vi "ex_subFileWrite.vi"(0 "Signals":dynamicdata(waveform), 1 "error in (no error)":errorcluster, 3 "Comment":string, 4 "Enable":bool=TRUE, 6 "new_file":bool, 7 "File Path in":path=path "c:/testdata.txt", 8 "File Dialog":bool, 9 "column headings":enum32{"one per segment", "once", "none"}(radio), 10 "Description":string, 11 "x_columns":enum32{"none", "one", "multiple"}(radio)=enum."multiple", 12 "multi_file":bool, 13 "fixed_width":bool=TRUE, 14 "serno_digits":i32=3, 15 "time_format_string":string="%Y-%m-%d_%H%M%S", 16 "overwrite_mode_multi":T6(ring)=enum."overwrite & backup", 17 "new_file_mode":u16(ring)=1 items=["Date & Time", "Serial No.", "Both"], 18 "overwrite_mode":T1(radio)=enum."overwrite & backup", 19 "new file options":T5, 20 "delimiter":string="\t", 22 "Reset":bool, 23 "Static File Path in":path=path "c:/testdata.txt", 24 "Lock file":bool, 25 "Simulate Non-First Call":bool, 26 "storage_format":T2, 27 "Ask each iteration":bool) -> (2 "error out":errorcluster, 5 "File Path out":path, 21 "Saving Data":bool)   [LabVIEW 2017]
uses:
  <vilib>/express/express output/ExFileWriteBlock.llb/ex_NewFileOptions.ctl
  <vilib>/express/express output/ExFileWriteBlock.llb/ex_WriteFileParams.ctl
  <vilib>/express/express input/ExFileReadBlock.llb/ex_ReadFileParams.ctl
  <vilib>/express/express shared/ExFile.llb/ex_FileFormats.ctl
panel:
  out "previous path":path
  in  "file params":T3={"delimiter"="\t", "origin time"=timestamp(0 s since 1904-01-01), "Flags"={"include col headings?"=TRUE, "x_columns"=0, "col headings always?"=TRUE, "time preference"=0, "hide col headings"=FALSE}, "Decimal Separator"=""} {"Flags"."time preference" items=["Absolute", "Relative"]; "Flags"."x_columns" items=["None", "One", "Multiple"]; "origin time" format="%<%X\n%x>T"}
  in  "1st":bool
  in  "File refnum":refnum<file>
  in  "origin time":timestamp format="%<%I:%M:%S %p\n%m/%d/%Y>T"
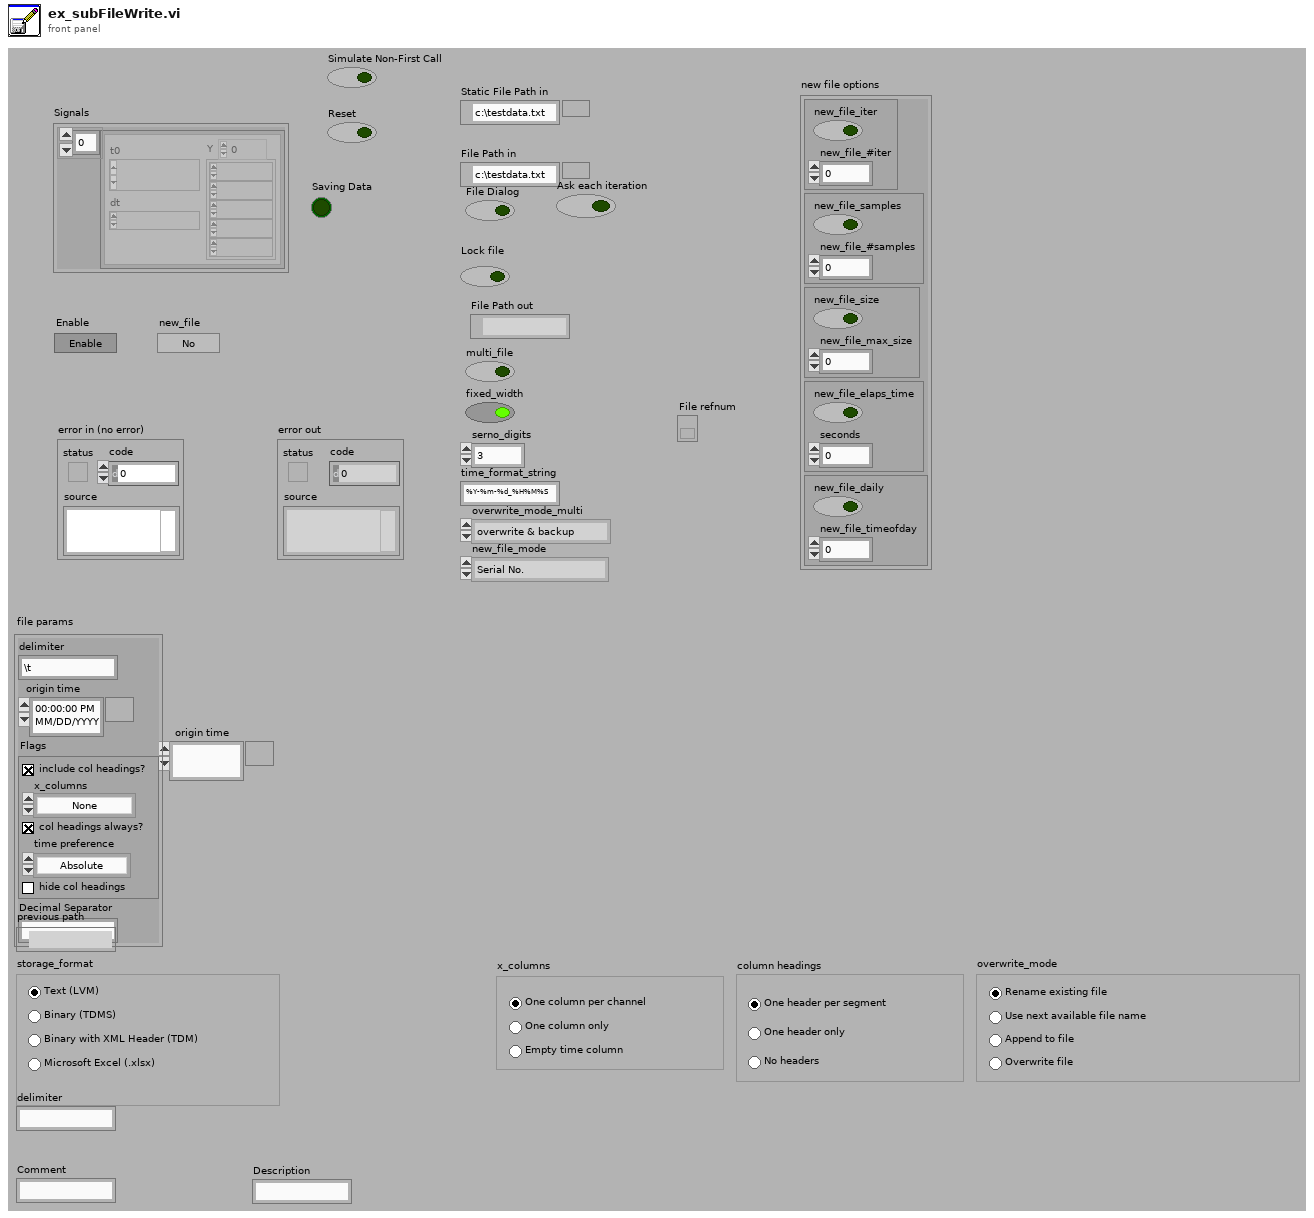
[diagram p1: front panel]
types:
  T1 = enum32{"overwrite", "overwrite & backup", "append", "next avail"}
  T2 = typedef "ex_FileFormats.ctl" = enum32{"lvm", "tdm", "tdms", "xlsx"}
  T3 = typedef "ex_WriteFileParams.ctl" = cluster{"delimiter":string, "origin time":timestamp, "Flags":T4, "Decimal Separator":string}
  T4 = typedef "ex_ReadFileParams.ctl" = cluster{"include col headings?":bool, "x_columns":u16, "col headings always?":bool, "time preference":u16, "hide col headings":bool}
  T5 = typedef "ex_NewFileOptions.ctl" = cluster{cluster{"new_file_iter":bool, "new_file_#iter":i32}, cluster{"new_file_samples":bool, "new_file_#samples":i32}, cluster{"new_file_size":bool, "new_file_max_size":i32}, cluster{"new_file_elaps_time":bool, "seconds":i32}, cluster{"new_file_daily":bool, "new_file_timeofday":i32}}
  T6 = enum16{"overwrite", "overwrite & backup", "next avail"}
  T7 = typedef "ex_userdefproperties.ctl" = cluster{"DAQmx Task":refnum<k21>, "User-defined properties":T8[], "Live values":variant[]}
  T8 = typedef "ex_userDefProperty.ctl" = cluster{"Name":string, "Object type":string, "usiDataType":T9, "propertySourceType":T10, "propertySource":string, "Value":variant, "ID":i32, "use def name":bool, "Source":string, "Built-in Prop":bool, "Attribute Type Enum":string[]}
  T9 = typedef "usiDataType.ctl" = enum16{"eNoTypeUsi", "eInt8Usi", "eInt16Usi", "eInt32Usi", "eInt64Usi", "eUInt8Usi", "eUInt16Usi", "eUInt32Usi", "eUInt64Usi", "eFloat32Usi", "eFloat64Usi", "- 0", "- 1", "- 2", "- 3", "- 4", "- 5", "- 6", "- 7", "- 8", "- 9", "eString8Usi", "eString16Usi", "eStringUsi", "eEnumUsi", "- 10", "- 11", "- 12", "- 13", "- 14", "eTimeUsi", "- 15", "- 16", "- 17", "- 18", "- 19", "- 20", "- 21", "- 22", "- 23", "eInstanceUsi", "eStoreUsi"}
  T10 = typedef "ex_propertySource.ctl" = enum16{"Manual", "System", "DAQmx Channel", "Terminal", "Ignore"}
  T11 = cluster{"file params":T3, "column headings":enum32{"one per segment", "once", "none"}, "origin time":timestamp, "File refnum":refnum<file>, "overwrite_mode_multi":enum16{"overwrite", "overwrite & backup", "next avail"}, "overwrite_mode":enum32{"overwrite", "overwrite & backup", "append", "next avail"}, "File Dialog":bool, "Description Out":string, "Comment Out":string, "serno_digits":i32, "fixed_width":bool, "new_file_mode":u16, "time_format_string":string, "multi_file":bool, "new file options":T5, "new_file":bool, "Simulate Non-First Call":bool}
  T12 = cluster{"channel\nrefnums":refnum<k20>[], "channel names":string[], "channel types":string[], "file refnum":refnum<k20>, "group refnum":refnum<k20>, "group name":string, "group type":string, "next T0":timestamp[], "dT":dbl[], "Start Time Stamp":timestamp, "channel length":u32[], "group index":u32, "group refnums":refnum<k20>[], "file name":string, "segment index":u32}
  T13 = typedef "ex_appendInfoTDM.ctl" = cluster{"channel\nrefnums":refnum<k20>[], "channel names":string[], "channel types":string[], "file refnum":refnum<k20>, "group refnum":refnum<k20>, "group name":string, "group type":string, "next T0":timestamp[], "dT":dbl[], "Start Time Stamp":timestamp, "channel length":u32[], "group index":u32, "group refnums":refnum<k20>[], "file name":string, "segment index":u32}
  T14 = cluster{"Start Timestamp":timestamp, "Timestamp":timestamp, "Relative Time?":bool, "X Dimension":string, "Signal Name":string, "Y Units":string, "X0":timestamp, "dX":dbl, "nPoints":i32}[]
  T15 = typedef "ex_WaveformAttribsPlus.ctl" = cluster{"Start Timestamp":timestamp, "Timestamp":timestamp, "Relative Time?":bool, "X Dimension":string, "Signal Name":string, "Y Units":string, "X0":timestamp, "dX":dbl, "nPoints":i32}
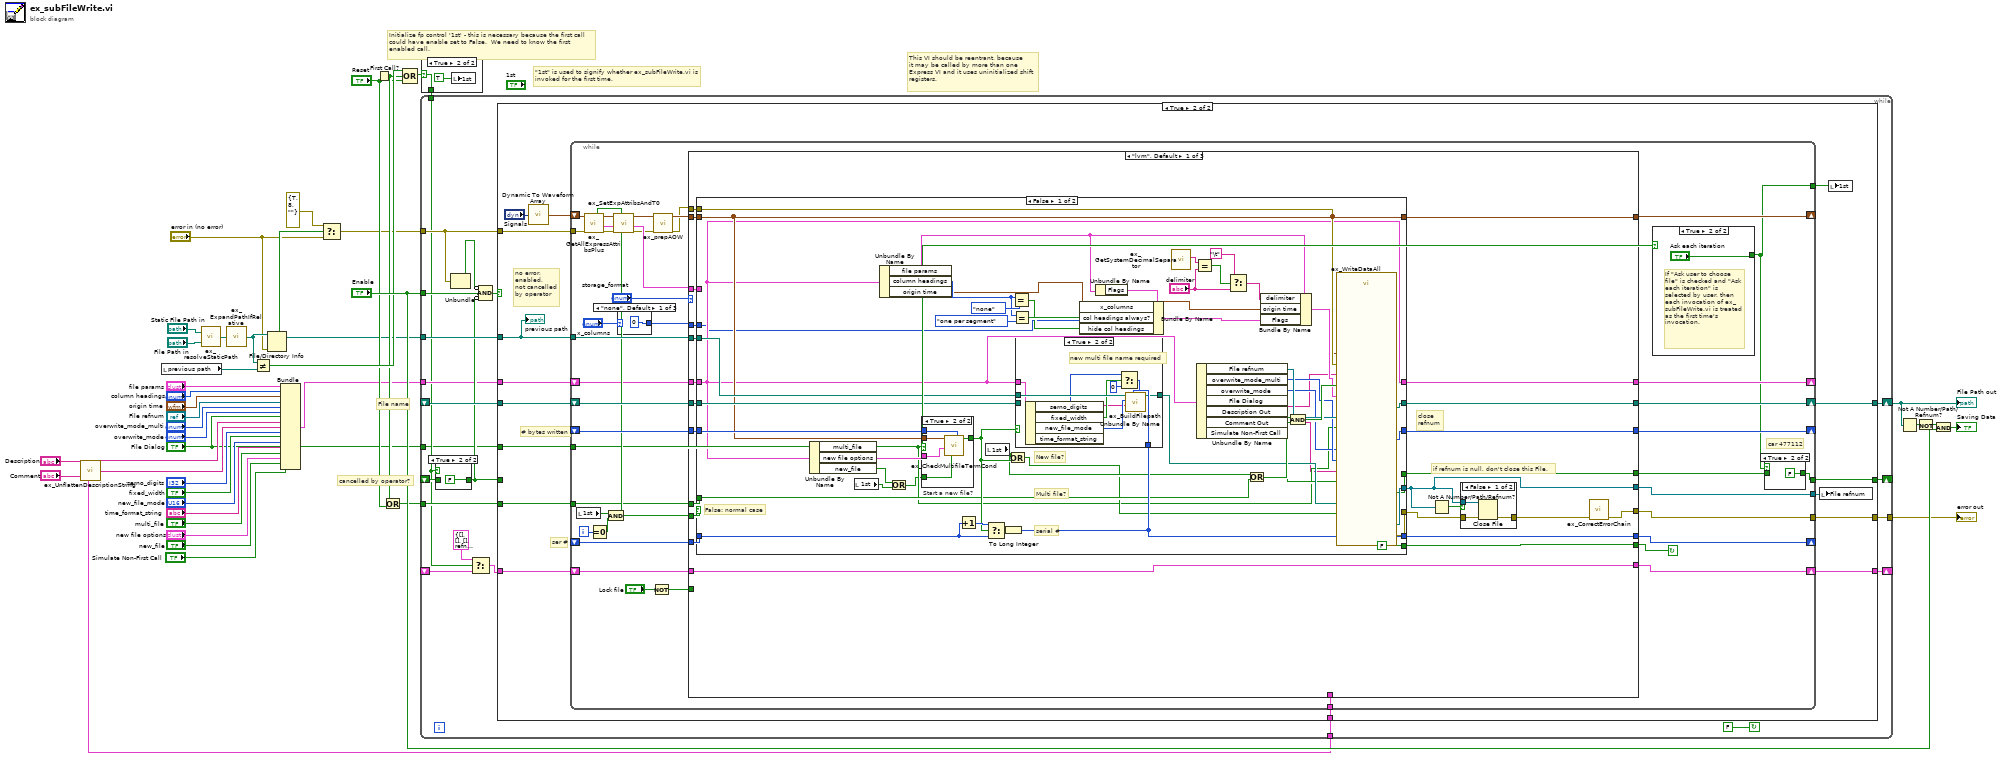
[diagram p0: block diagram]
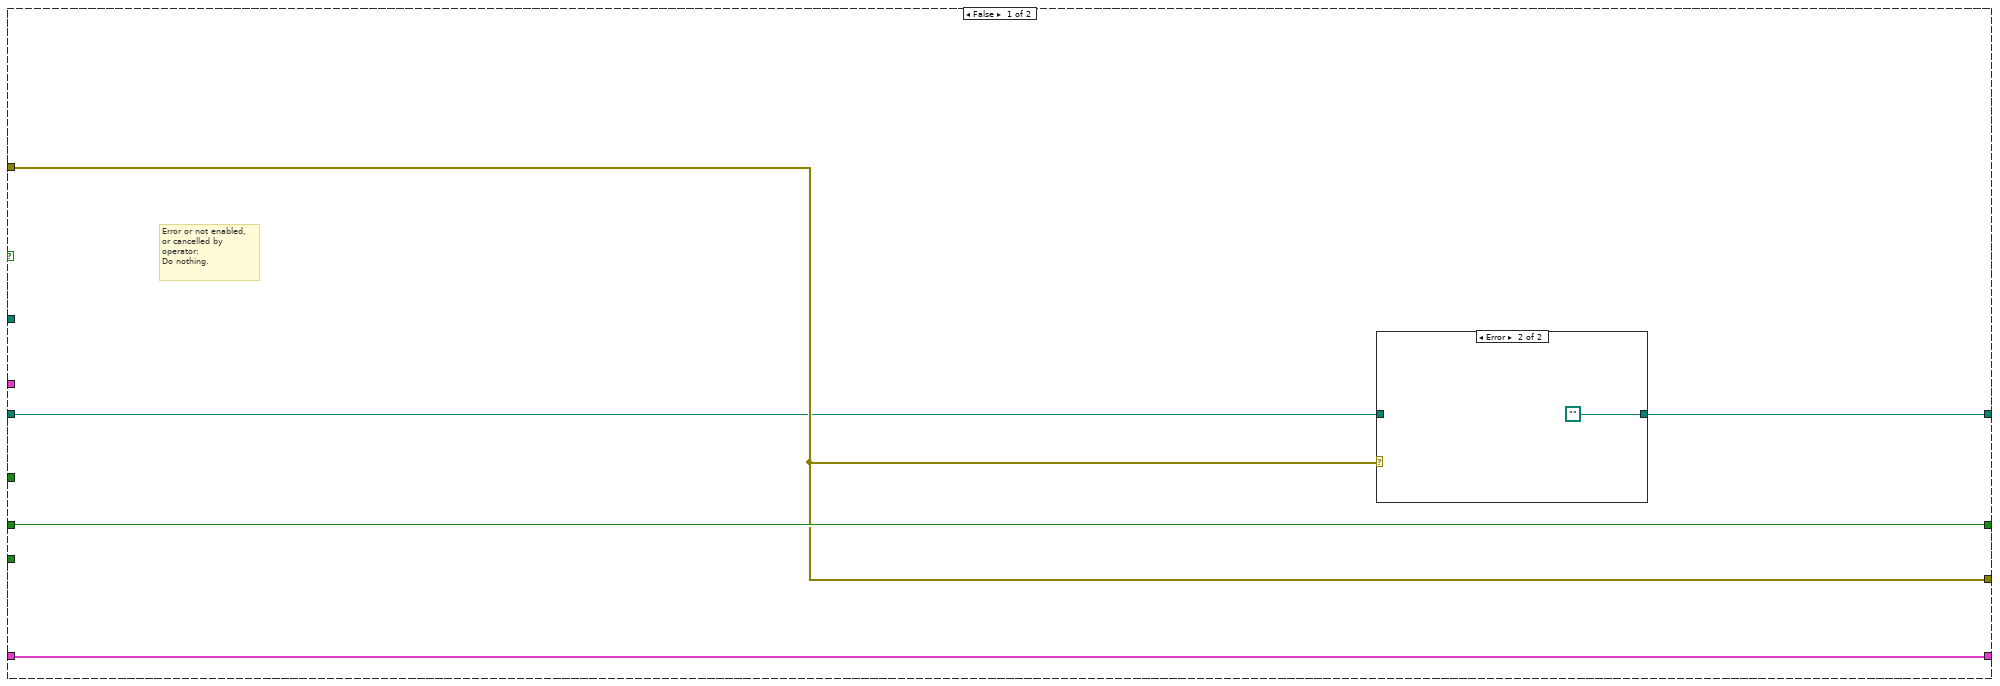
[diagram p3: hidden frame]
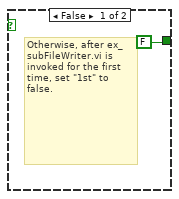
[diagram p6: hidden frame]
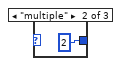
[diagram p7: hidden frame]
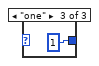
[diagram p8: hidden frame]
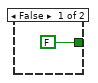
[diagram p11: hidden frame]
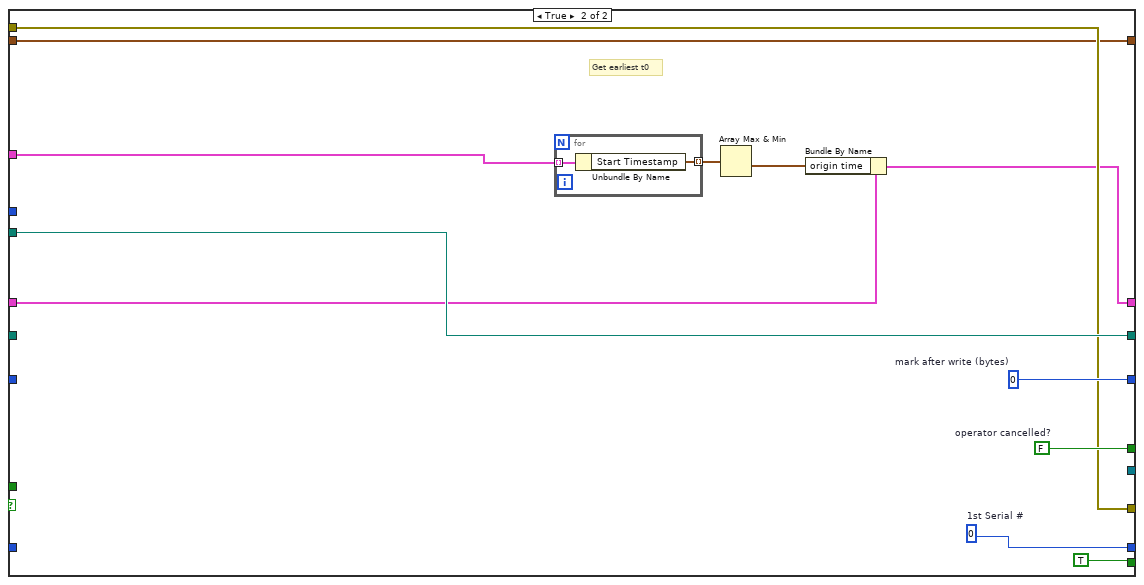
[diagram p12: hidden frame]
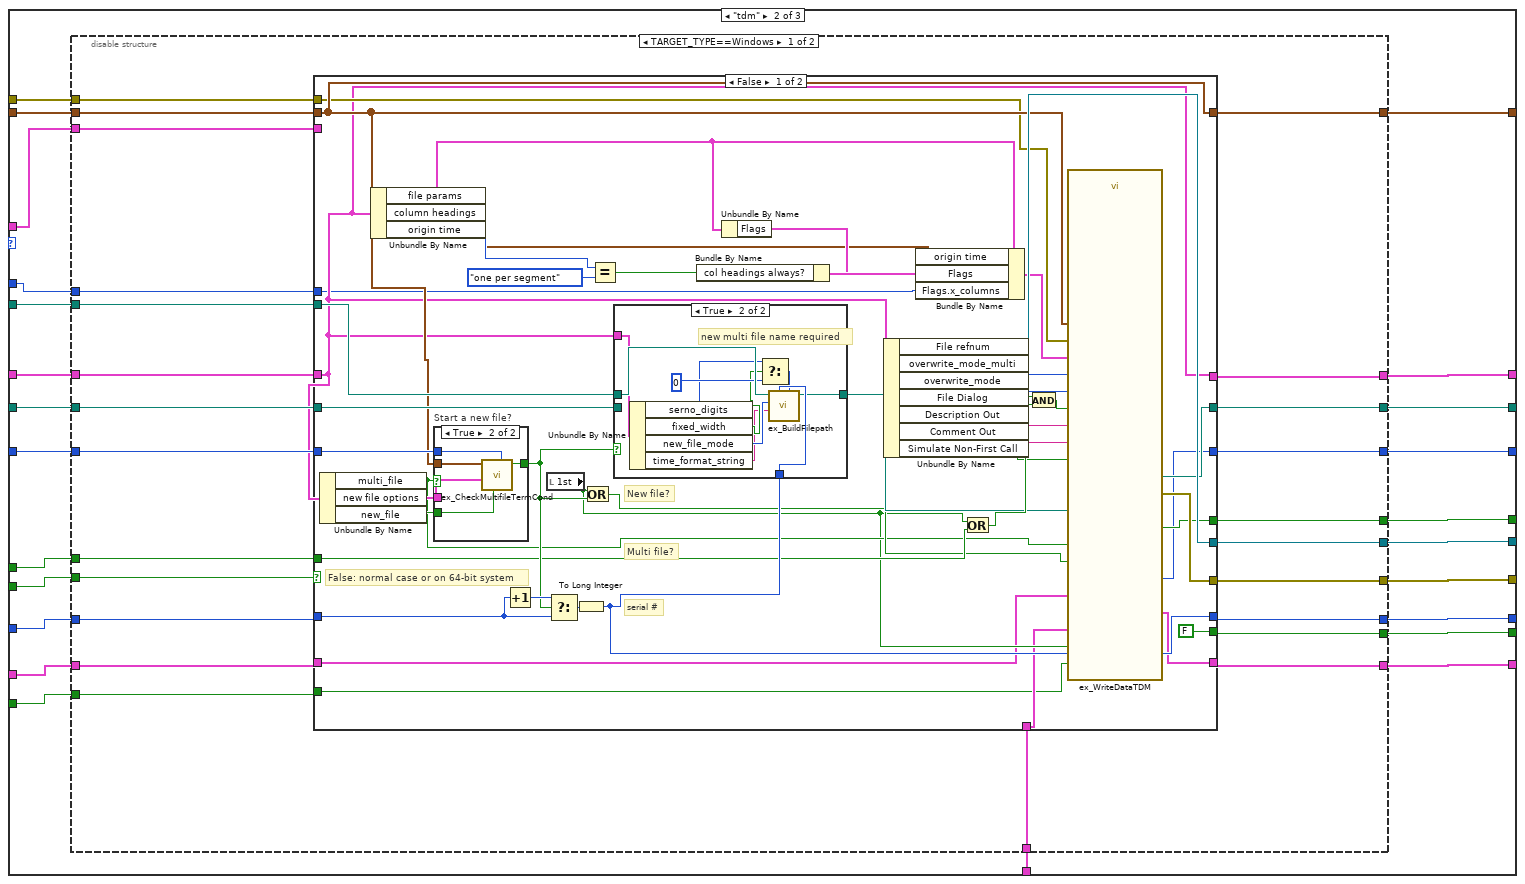
[diagram p13: hidden frame]
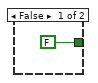
[diagram p15: hidden frame]
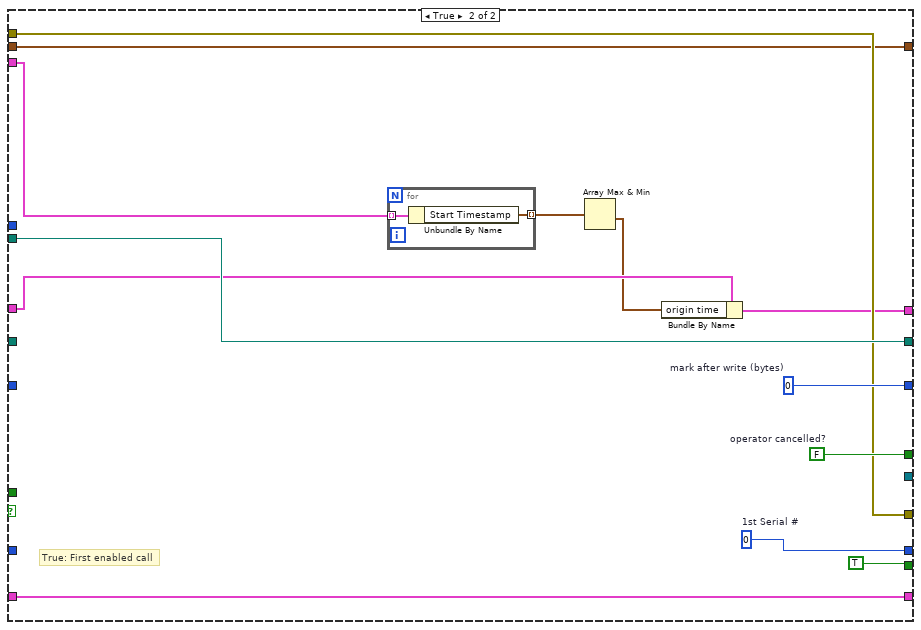
[diagram p16: hidden frame]
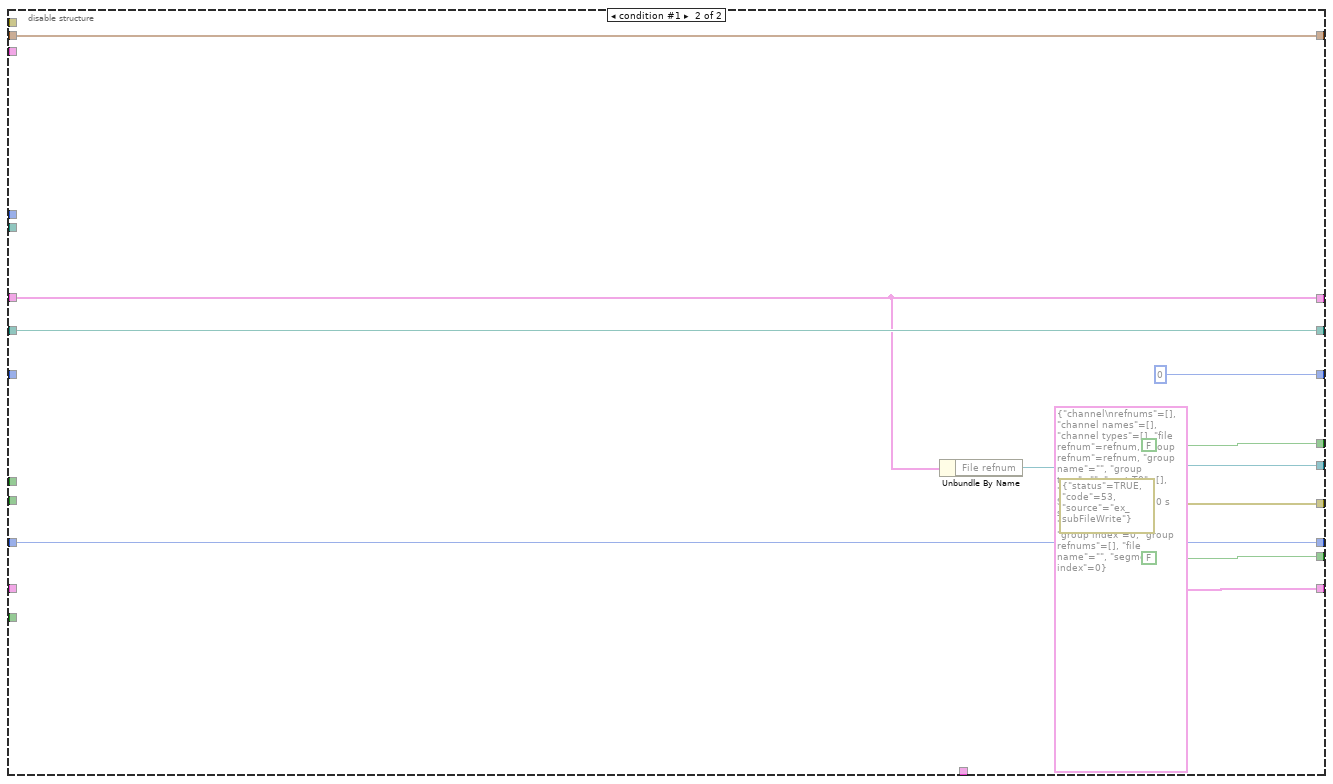
[diagram p17: hidden frame]
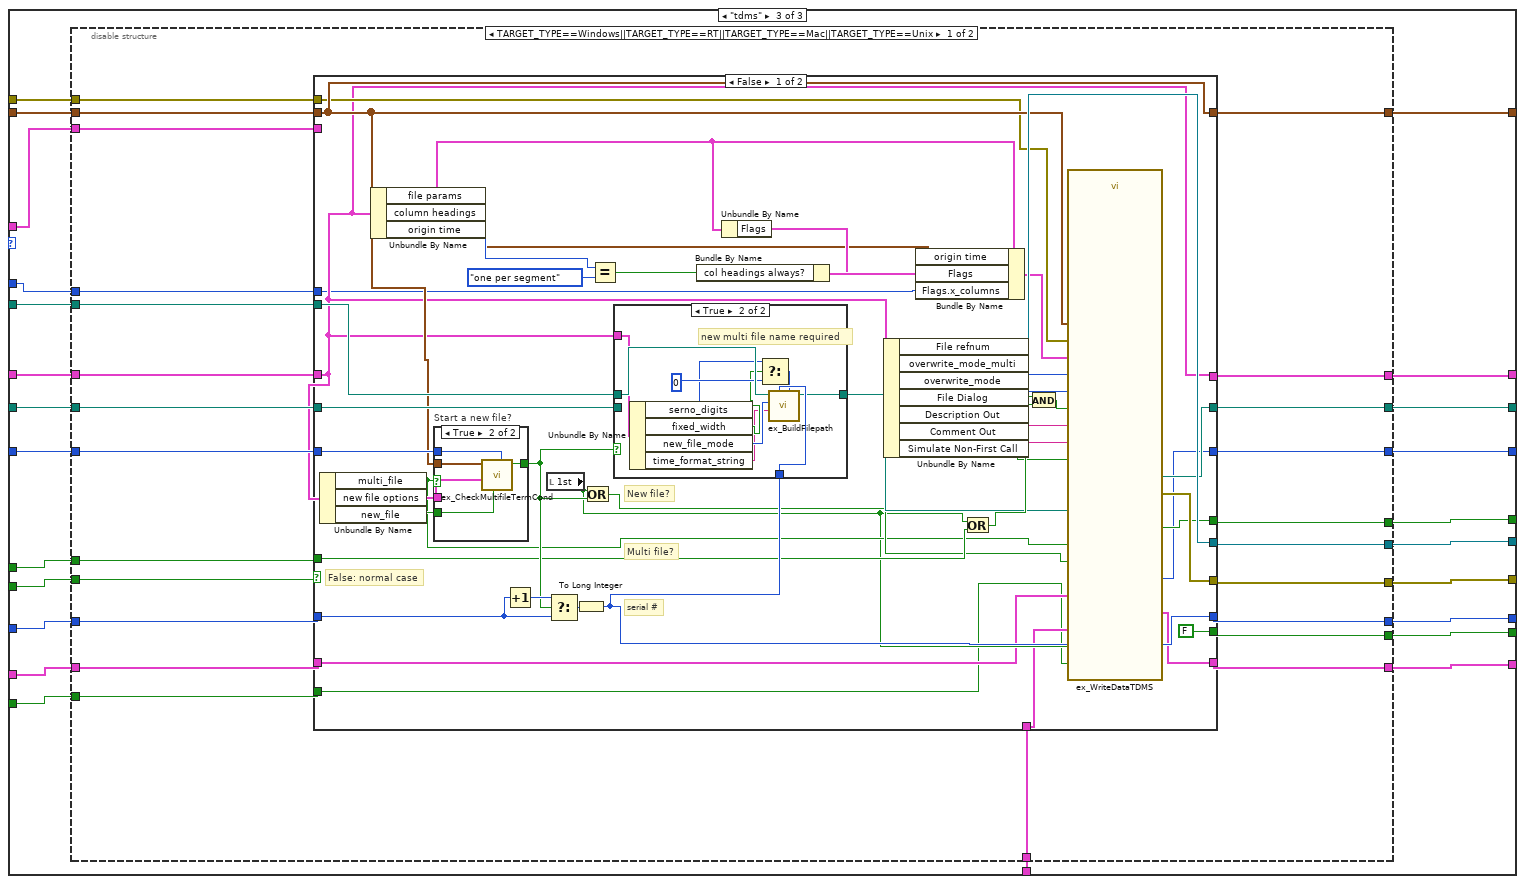
[diagram p18: hidden frame]
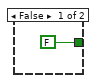
[diagram p20: hidden frame]
diagram:
  # "\"1st\" is used to signify whether ex_subFileWrite.vi is invoked for the first time."
  # "File name"
  # "This VI should be reentrant, because\nit may be called by more than one\nExpress VI and it uses uninitialized shift \nregisters."
  # "cancelled by operator?"
  # "Initialize fp control '1st' - this is necessary because the first call\ncould have enable set to False.  We need to know the first\nenabled call."
  n1 = call <vilib>:"ex_UnflattenDescriptionString.vi"("Description"="Description", "Comment"="Comment") -> ("Description Out"=w6:string, "Comment Out"=w5:string, "DAQmx Task"=w4:T7)
  n2 = local read "previous path"() -> (w36:path)
  n3 = call <vilib>:"ex_resolveStaticPath.vi"("file path in"="File Path in", "static path in"="Static File Path in") -> ("Path"=w13:path)
  n4 = call <vilib>:"ex_ExpandPathIfRelative.vi"("Path"=w13) -> ("Expanded path"=w12:path)  [unwired: 4 out]
  n5 = Not Equal?(x=w12, y=w36) -> (x != y?=w34:bool)
  n6 = File/Directory Info(path=w12, error in="error in (no error)") -> (path out=w11:path, directory=w9:bool)  [unwired: 5 out]
  n7 = Bundle("file params"="file params", "column headings"="column headings", "origin time"="origin time", "File refnum"="File refnum", "overwrite_mode_multi"="overwrite_mode_multi", "overwrite_mode"="overwrite_mode", "File Dialog"="File Dialog", "Description Out"=w6, "Comment Out"=w5, "serno_digits"="serno_digits", "fixed_width"="fixed_width", "new_file_mode"="new_file_mode", "time_format_string"="time_format_string", "multi_file"="multi_file", "new file options"="new file options", "new_file"="new_file", "Simulate Non-First Call"="Simulate Non-First Call") -> (w14:T11)  [unwired: 1 out]
  n8 = Select(t=errorcluster {"status"=TRUE, "code"=8, "source"=""}, s=w9, f="error in (no error)") -> (s? t:f=w10:errorcluster)
  n9 = First Call?() -> (First Call?: T/F=w33:bool)
  n10 = Or(x=w33, y="Reset") -> (x .or. y?=w31:bool)
  n11 = Compound Arithmetic op=OR(w34, w33, "Reset") -> (w35:bool)
  n12 = case shown="False" w35 {
    selector: w35 -> [w44 w45]
    tunnel: [w44 w45] -> w43
    frame False {
    }
    frame True {
      n13 = local write "1st"(TRUE ("1st")) -> ()
    }
  }
  n14 = while {
    tunnel: [w67] -> w30
    tunnel: w43 -> [w48]
    tunnel: w10 -> [w65]
    shift-right: [w63] -> _
    shift-left: _ -> [w62]
    shift-right: [w60] -> w29
    shift-left: _ -> [w61]
    tunnel: "Enable" -> [w59]
    tunnel: w11 -> [w58]
    tunnel: w31 -> [w55]
    tunnel: w14 -> [w54]
    shift-right: [w53] -> _
    shift-left: _ -> [w50]
    tunnel: w4 -> [w52]
    tunnel: "File Dialog" -> [w47]
    stop <- FALSE continue-if-true
    n15 = case shown="True" w48 {
      tunnel: w62 -> [w68 _]
      tunnel: [w68 FALSE ("operator cancelled?")] -> w56
      frame False {
      }
      frame True {
      }
    }
    n16 = Unbundle(w65) -> ("status"=w57:bool)  [unwired: 2 out]
    n17 = Select(t=T12 {"channel\nrefnums"=[], "channel names"=[], "channel types"=[], "file refnum"=refnum, "group refnum"=refnum, "group name"="", "group type"="", "next T0"=[], "dT"=[], "Start Time Stamp"=timestamp(0 s since 1904-01-01), "channel length"=[], "group index"=0, "group refnums"=[], "file name"="", "segment index"=0} ("append info out"), s=w48, f=w50) -> (s? t:f=w49:T13)
    n18 = Compound Arithmetic op=AND(invert w57, w59, invert w56) -> (w66:bool)
    n19 = case shown="True" w66 {
      tunnel: [w72 w83] -> w67
      tunnel: w65 -> [w72 w92]
      tunnel: [w74 w91] -> w63
      tunnel: w56 -> [w74 _]
      tunnel: [w71 w90] -> w60
      tunnel: w61 -> [w70 w89]
      tunnel: w58 -> [_ w80]
      tunnel: w55 -> [_ w87]
      tunnel: w54 -> [_ w85]
      tunnel: [w73 w82] -> w53
      tunnel: w49 -> [w73 w81]
      tunnel: w52 -> [_ w79]
      tunnel: w47 -> [_ w77]
      frame False {
        # "Error or not enabled,\nor cancelled by\noperator:\nDo nothing."
        n20 = case shown="No Error" w72 {
          tunnel: [w75 path ""] -> w71
          tunnel: w70 -> [w75 _]
          frame No Error {
          }
          frame Error {
          }
        }
      }
      frame True {
        # "no error,\nenabled,\nnot cancelled\nby operator"
        # "# bytes written"
        # "ser #"
        n21 = call <vilib>:"Dynamic To Waveform Array.vi"("Input"="Signals") -> ("Output"=w84:waveform(dbl)[])  [unwired: 4 out]
        n22 = while {
          tunnel: w92 -> [w121]
          shift-right: [w130] -> _
          shift-left: _ -> [w129]
          tunnel: [w132] -> w83
          shift-right: [w122] -> w90
          shift-left: w89 -> [w128]
          shift-right: [w124] -> _
          shift-left: _ -> [w131]
          tunnel: [w127] -> w86
          tunnel: w80 -> [w123]
          tunnel: [w93] -> w91
          shift-right: [w120] -> _
          shift-left: w84 -> [w109]
          tunnel: w87 -> [w112]
          shift-right: [w108] -> _
          shift-left: w85 -> [w110]
          shift-right: [w107] -> w82
          shift-left: w81 -> [w106]
          tunnel: w79 -> [w99]
          tunnel: [w95] -> w78
          tunnel: w77 -> [w96]
          i -> [w126]
          stop <- w133 continue-if-true
          # "car 477112"
          n23 = local read "1st"() -> (w113:bool)
          n24 = call <vilib>:"ex_GetAllExpressAttribsPlus.vi"("error in"=w121, "Signals in"=w109) -> ("error out"=w115:errorcluster, "All Express Wave Attributes Plus"=w114:T14, "Signals out"=w118:waveform(dbl)[], "Time Attribs Not Found"=w116:bool[])  [unwired: 1 in, 5 out]
          n25 = Equal To 0?(x=w126) -> (x = 0?=w125:bool)
          n26 = And(x=w113, y=w125) -> (x .and. y?=w119:bool)
          n27 = call <vilib>:"ex_SetExpAttribsAndT0.vi"("Latch Origin TS? (T)"=w119, "Set? (T if empty)"=w116, "error in (no error)"=w115, "Express Attributes Plus in"=w114, "Signals"=w118) -> ("error out"=w101:errorcluster, "Express Wave Attributes Plus out"=w117:T15[], "Signals With Attributes"=w103:waveform(dbl)[])  [unwired: 1 in, 3 out]
          n28 = case shown="\"none\", Default" "x_columns" {
            tunnel: [u16 0 ("x_columns") u16 2 ("x_columns") u16 1 ("x_columns")] -> w104
            frame "none", Default {
            }
            frame "multiple" {
            }
            frame "one" {
            }
          }
          n29 = Not(x="Lock file") -> (.not. x?=w97:bool)
          n30 = call <vilib>:"ex_prepAOW.vi"("error in (no error)"=w101, "Dynamic Data"=w103) -> ("error out"=w100:errorcluster, 3:w102:waveform(dbl)[])  [unwired: 1 in, 3 out]
          n31 = case shown="\"lvm\", Default" "storage_format" {
            tunnel: [w164 w274 w409] -> w133
            tunnel: [w148 w273 w408] -> w132
            tunnel: w131 -> [w163 w272 w407]
            tunnel: [w162 w271 w406] -> w130
            tunnel: w129 -> [w161 w270 w405]
            tunnel: w128 -> [w160 w269 w404]
            tunnel: [w141 w258 w393] -> w127
            tunnel: [w159 w268 w403] -> w124
            tunnel: w123 -> [w158 w267 w402]
            tunnel: [w157 w266 w401] -> w94
            tunnel: [w156 w265 w400] -> w122
            tunnel: [w155 w264 w399] -> w120
            tunnel: w119 -> [w154 w263 w398]
            tunnel: w102 -> [w153 w257 w392]
            tunnel: w100 -> [w152 w262 w397]
            tunnel: w117 -> [w151 w261 w396]
            tunnel: w112 -> [w150 w260 w395]
            tunnel: w110 -> [w149 w259 w394]
            tunnel: [w147 w256 w391] -> w108
            tunnel: [w146 w255 w390] -> w107
            tunnel: w106 -> [w146 w254 w389]
            tunnel: w104 -> [w145 w253 w388]
            tunnel: w99 -> [_ w252 w387]
            tunnel: w97 -> [_ w251 w386]
            frame "lvm", Default {
              # "if refnum is null, don't close this File."
              # "close\nrefnum"
              n32 = case shown="False" w154 {
                tunnel: [FALSE TRUE] -> w164
                tunnel: [w192 _] -> w141
                tunnel: [w189 w241] -> w144
                tunnel: [w190 w248] -> w159
                tunnel: w163 -> [w212 _]
                tunnel: w152 -> [w208 w241]
                tunnel: [w217 w246] -> w162
                tunnel: [w191 w247] -> w156
                tunnel: w161 -> [w218 _]
                tunnel: w160 -> [w214 _]
                tunnel: w153 -> [w182 w240]
                tunnel: w158 -> [w211 w247]
                tunnel: [w183 w244] -> w157
                tunnel: w151 -> [_ w242]
                tunnel: [w182 w240] -> w155
                tunnel: w150 -> [w201 _]
                tunnel: w149 -> [w180 w239]
                tunnel: [w180 w237] -> w147
                tunnel: w145 -> [w179 _]
                frame False {
                  # "Multi file?"
                  # "New file?"
                  # "False: normal case"
                  # "serial #"
                  n33 = Unbundle By Name(w180) -> ("multi_file"=w184:bool, "new file options"=w193:T5, "new_file"=w171:bool)
                  n34 = local read "1st"() -> (w170:bool)
                  n35 = Unbundle By Name(w180) -> ("file params"=w199:T3, "column headings"=w198:enum32{"one per segment", "once", "none"}, "origin time"=w181:timestamp)
                  n36 = Or(x=w171, y=w170) -> (x .or. y?=w169:bool)
                  n37 = case "Start a new file?" shown="True" w184 {
                    tunnel: [FALSE ("start new file?") w236] -> w213
                    tunnel: w182 -> [_ w235]
                    tunnel: w212 -> [_ w234]
                    tunnel: w193 -> [_ w233]
                    tunnel: w169 -> [_ w232]
                    frame False {
                    }
                    frame True {
                      n38 = call <vilib>:"ex_CheckMultifileTermCond.vi"("file size (bytes)"=w234, "new_file_now"=w232, "termination conditions"=w233, "Signals"=w235) -> ("start new file?"=w236:bool)  [unwired: 7 out]
                    }
                  }
                  n39 = Increment(x=w218) -> (x+1=w219:i32)
                  n40 = local read "1st"() -> (w200:bool)
                  n41 = Select(t=w219, s=w213, f=w218) -> (s? t:f=w216:i32)
                  n42 = To Long Integer(number=w216) -> (32bit integer=w217:i32)
                  n43 = Or(x=w200, y=w213) -> (x .or. y?=w185:bool)
                  n44 = Equal?(x=w198, y=enum16{"one per segment", "once", "none"}."none") -> (x = y?=w204:bool)
                  n45 = Equal?(x=w198, y=enum16{"one per segment", "once", "none"}."one per segment") -> (x = y?=w205:bool)
                  n46 = case shown="True" w213 {
                    tunnel: w217 -> [_ w230]
                    tunnel: [w220 w229] -> w188
                    tunnel: w214 -> [w220 _]
                    tunnel: w211 -> [_ w228]
                    tunnel: w180 -> [_ w225]
                    frame False {
                      # "No new file - use old file name"
                    }
                    frame True {
                      # "new multi file name required"
                      n47 = Unbundle By Name(w225) -> ("serno_digits"=w224:i32, "fixed_width"=w223:bool, "new_file_mode"=w222:u16, "time_format_string"=w221:string)
                      n48 = Select(t=w224, s=w223, f=0) -> (s? t:f=w226:i32)
                      n49 = call <vilib>:"ex_BuildFilepath.vi"("serial digits"=w226, "serial num"=w230, "time format string"=w221, "naming mode"=w222, "name base"=w228) -> ("built name"=w229:path)  [unwired: 1 in, 5 out]
                    }
                  }
                  n50 = Unbundle By Name(w199) -> ("Flags"=w209:T4)
                  n51 = Bundle By Name(cluster=w209, "x_columns"=w179, "col headings always?"=w205, "hide col headings"=w204) -> (w210:T4)
                  n52 = call <vilib>:"ex_GetSystemDecimalSeparator.vi"() -> ("Decimal Seperator"=w176:string)  [unwired: 11 out]
                  n53 = Equal?(x=w176, y="delimiter") -> (x = y?=w175:bool)
                  n54 = Unbundle By Name(w180) -> ("File refnum"=w197:refnum<file>, "overwrite_mode_multi"=w196:T6, "overwrite_mode"=w195:T1, "File Dialog"=w194:bool, "Description Out"=w177:string, "Comment Out"=w178:string, "Simulate Non-First Call"=w187:bool)
                  n55 = Select(t="\t", s=w175, f="delimiter") -> (s? t:f=w172:string)
                  n56 = Or(x=w200, y=w201) -> (x .or. y?=w203:bool)
                  n57 = Bundle By Name(cluster=w199, "delimiter"=w172, "origin time"=w181, "Flags"=w210) -> (w186:T3)
                  n58 = And(x=w194, y=w203) -> (x .and. y?=w202:bool)
                  n59 = call <vilib>:"ex_WriteDataAll.vi"("file path"=w188, "File refnum in"=w197, "Signals"=w182, "overwrite_mode_multi"=w196, "overwrite_mode"=w195, "error in (no error)"=w208, "file dialog?"=w202, "Description"=w177, "multi_file"=w184, "Comment"=w178, "new file?"=w185, "Simulate Non-First Call"=w187, "file params"=w186) -> ("operator cancelled?"=w183:bool, "file path out"=w191:path, "refnum out"=w192:refnum<file>, "mark after write (bytes)"=w190:i32, "error out"=w189:errorcluster)  [unwired: 2 out]
                }
                frame True {
                  w244 = FALSE  # operator cancelled?
                  w248 = 0  # mark after write (bytes)
                  w246 = 0  # 1st Serial #
                  # "True: First enabled call"
                  # "Get earliest t0"
                  n60 = for {
                    tunnel: w242 -> [w250] mode=indexing
                    tunnel: [w249] -> w243 mode=indexing
                    n61 = Unbundle By Name(w250) -> ("Start Timestamp"=w249:timestamp)
                  }
                  n62 = Array Max & Min(array=w243) -> (min value=w238:timestamp)  [unwired: 3 out]
                  n63 = Bundle By Name(cluster=w239, "origin time"=w238) -> (w237:T11)
                }
              }
              n64 = Not A Number/Path/Refnum?(number/path/refnum=w141) -> (NaN/Path/Refnum?=w142:bool)
              n65 = case shown="False" w142 {
                tunnel: w144 -> [w167 w168]
                tunnel: [w166 w168] -> w143
                tunnel: w141 -> [w165 _]
                frame False {
                  n66 = Close File(refnum=w165, error in=w167) -> (error out=w166:errorcluster)  [unwired: 1 out]
                }
                frame True {
                }
              }
              n67 = call <vilib>:"ex_CorrectErrorChain.vi"("error in (no error)"=w143) -> ("error out"=w148:errorcluster)  [unwired: 1 in, 9 out]
            }
            frame "tdm" {
              n68 = disable-structure shown="TARGET_TYPE==Windows" {
                disable-tunnel: [w298 FALSE] -> w274
                disable-tunnel: [w297 errorcluster {"status"=TRUE, "code"=53, "source"="ex_subFileWrite"} ("error out")] -> w273
                disable-tunnel: w272 -> [w296 _]
                disable-tunnel: [w295 w380] -> w271
                disable-tunnel: w270 -> [w294 w380]
                disable-tunnel: w269 -> [w293 w385]
                disable-tunnel: [w292 0 ("mark after write (bytes)")] -> w268
                disable-tunnel: w267 -> [w291 _]
                disable-tunnel: [w290 FALSE ("operator cancelled?")] -> w266
                disable-tunnel: [w289 w385] -> w265
                disable-tunnel: [w288 w384] -> w264
                disable-tunnel: w263 -> [w275 _]
                disable-tunnel: w262 -> [w287 _]
                disable-tunnel: w261 -> [w286 _]
                disable-tunnel: w260 -> [w276 _]
                disable-tunnel: w259 -> [w285 w383]
                disable-tunnel: [w284 w382] -> w258
                disable-tunnel: w257 -> [w283 w384]
                disable-tunnel: [w282 w383] -> w256
                disable-tunnel: [w281 T12 {"channel\nrefnums"=[], "channel names"=[], "channel types"=[], "file refnum"=refnum, "group refnum"=refnum, "group name"="", "group type"="", "next T0"=[], "dT"=[], "Start Time Stamp"=timestamp(0 s since 1904-01-01), "channel length"=[], "group index"=0, "group refnums"=[], "file name"="", "segment index"=0} ("append info out")] -> w255
                disable-tunnel: w254 -> [w280 _]
                disable-tunnel: w253 -> [w279 _]
                disable-tunnel: w252 -> [w278 _]
                disable-tunnel: w251 -> [w277 _]
                frame condition #0 (active) {
                  n69 = case shown="False" w275 {
                    tunnel: [FALSE TRUE] -> w298
                    tunnel: [w308 w368] -> w297
                    tunnel: [w306 w373] -> w292
                    tunnel: w296 -> [w336 _]
                    tunnel: w287 -> [w321 w368]
                    tunnel: [w341 w371] -> w295
                    tunnel: [w309 w372] -> w289
                    tunnel: w294 -> [w342 _]
                    tunnel: w293 -> [w338 _]
                    tunnel: w291 -> [w335 w372]
                    tunnel: [w307 w369] -> w290
                    tunnel: w286 -> [_ w366]
                    tunnel: [w322 w367] -> w288
                    tunnel: w276 -> [w329 _]
                    tunnel: w285 -> [w319 w364]
                    tunnel: [w323 _] -> w284
                    tunnel: w283 -> [w322 w367]
                    tunnel: [w319 w362] -> w282
                    tunnel: [w305 w361] -> w281
                    tunnel: w280 -> [w304 w361]
                    tunnel: w279 -> [w318 _]
                    tunnel: w278 -> [w303 _]
                    tunnel: w277 -> [w299 _]
                    frame False {
                      # "Multi file?"
                      # "New file?"
                      # "False: normal case or on 64-bit system"
                      # "serial #"
                      n70 = Unbundle By Name(w319) -> ("multi_file"=w311:bool, "new file options"=w325:T5, "new_file"=w324:bool)
                      n71 = Unbundle By Name(w319) -> ("file params"=w328:T3, "column headings"=w327:enum32{"one per segment", "once", "none"}, "origin time"=w320:timestamp)
                      n72 = case "Start a new file?" shown="True" w311 {
                        tunnel: [FALSE ("start new file?") w360] -> w337
                        tunnel: w322 -> [_ w359]
                        tunnel: w336 -> [_ w358]
                        tunnel: w325 -> [_ w357]
                        tunnel: w324 -> [_ w356]
                        frame False {
                        }
                        frame True {
                          n73 = call <vilib>:"ex_CheckMultifileTermCond.vi"("file size (bytes)"=w358, "new_file_now"=w356, "termination conditions"=w357, "Signals"=w359) -> ("start new file?"=w360:bool)  [unwired: 7 out]
                        }
                      }
                      n74 = Increment(x=w342) -> (x+1=w343:i32)
                      n75 = local read "1st"() -> (w310:bool)
                      n76 = Select(t=w343, s=w337, f=w342) -> (s? t:f=w340:i32)
                      n77 = To Long Integer(number=w340) -> (32bit integer=w341:i32)
                      n78 = Or(x=w310, y=w337) -> (x .or. y?=w312:bool)
                      n79 = Equal?(x=w327, y=enum16{"one per segment", "once", "none"}."one per segment") -> (x = y?=w331:bool)
                      n80 = case shown="True" w337 {
                        tunnel: w341 -> [_ w354]
                        tunnel: [w344 w353] -> w313
                        tunnel: w338 -> [w344 _]
                        tunnel: w335 -> [_ w352]
                        tunnel: w319 -> [_ w349]
                        frame False {
                          # "No new file - use old file name"
                        }
                        frame True {
                          # "new multi file name required"
                          n81 = Unbundle By Name(w349) -> ("serno_digits"=w348:i32, "fixed_width"=w347:bool, "new_file_mode"=w346:u16, "time_format_string"=w345:string)
                          n82 = Select(t=w348, s=w347, f=0) -> (s? t:f=w350:i32)
                          n83 = call <vilib>:"ex_BuildFilepath.vi"("serial digits"=w350, "serial num"=w354, "time format string"=w345, "naming mode"=w346, "name base"=w352) -> ("built name"=w353:path)  [unwired: 1 in, 5 out]
                        }
                      }
                      n84 = Unbundle By Name(w328) -> ("Flags"=w333:T4)
                      n85 = Bundle By Name(cluster=w333, "col headings always?"=w331) -> (w334:T4)
                      n86 = Unbundle By Name(w319) -> ("File refnum"=w323:refnum<file>, "overwrite_mode_multi"=w316:T6, "overwrite_mode"=w315:T1, "File Dialog"=w326:bool, "Description Out"=w301:string, "Comment Out"=w300:string, "Simulate Non-First Call"=w302:bool)
                      n87 = Bundle By Name(cluster=w328, "origin time"=w320, "Flags"=w334, "Flags.x_columns"=w318) -> (w317:T3)
                      n88 = Or(x=w310, y=w329) -> (x .or. y?=w330:bool)
                      n89 = And(x=w326, y=w330) -> (x .and. y?=w314:bool)
                      n90 = call <vilib>:"ex_WriteDataTDM.vi"("file path"=w313, "first call"=w310, "Lock file"=w299, "Signals"=w322, "overwrite_mode_multi"=w316, "overwrite_mode"=w315, "error in (no error)"=w321, "file dialog?"=w314, "Description"=w301, "multi_file"=w311, "Comment"=w300, "new file?"=w312, "Simulate Non-First Call"=w302, "file params"=w317, "append info"=w304, "DAQmx Task"=w303) -> ("operator cancelled?"=w307:bool, "file path out"=w309:path, "bytes written"=w306:i32, "append info out"=w305:T13, "error out"=w308:errorcluster)  [unwired: 7 out]
                    }
                    frame True {
                      w369 = FALSE  # operator cancelled?
                      w373 = 0  # mark after write (bytes)
                      w371 = 0  # 1st Serial #
                      # "True: First enabled call"
                      n91 = for {
                        tunnel: w366 -> [w375] mode=indexing
                        tunnel: [w374] -> w365 mode=indexing
                        n92 = Unbundle By Name(w375) -> ("Start Timestamp"=w374:timestamp)
                      }
                      n93 = Array Max & Min(array=w365) -> (min value=w363:timestamp)  [unwired: 3 out]
                      n94 = Bundle By Name(cluster=w364, "origin time"=w363) -> (w362:T11)
                    }
                  }
                }
                frame condition #1 {
                  n95 = Unbundle By Name(w383) -> ("File refnum"=w382:refnum<file>)
                }
              }
            }
            frame "tdms" {
              n96 = disable-structure shown="TARGET_TYPE==Windows||TARGET_TYPE==RT||TARGET_TYPE==Mac||TARGET_TYPE==Unix" {
                disable-tunnel: [w433 FALSE] -> w409
                disable-tunnel: [w432 errorcluster {"status"=TRUE, "code"=53, "source"="ex_subFileWrite"} ("error out")] -> w408
                disable-tunnel: w407 -> [w431 _]
                disable-tunnel: [w430 w515] -> w406
                disable-tunnel: w405 -> [w429 w515]
                disable-tunnel: w404 -> [w428 w520]
                disable-tunnel: [w427 0 ("mark after write (bytes)")] -> w403
                disable-tunnel: w402 -> [w426 _]
                disable-tunnel: [w425 FALSE ("operator cancelled?")] -> w401
                disable-tunnel: [w424 w520] -> w400
                disable-tunnel: [w423 w519] -> w399
                disable-tunnel: w398 -> [w422 _]
                disable-tunnel: w397 -> [w421 _]
                disable-tunnel: w396 -> [w420 _]
                disable-tunnel: w395 -> [w419 _]
                disable-tunnel: w394 -> [w418 w518]
                disable-tunnel: [w417 w517] -> w393
                disable-tunnel: w392 -> [w416 w519]
                disable-tunnel: [w415 w518] -> w391
                disable-tunnel: [w414 T12 {"channel\nrefnums"=[], "channel names"=[], "channel types"=[], "file refnum"=refnum, "group refnum"=refnum, "group name"="", "group type"="", "next T0"=[], "dT"=[], "Start Time Stamp"=timestamp(0 s since 1904-01-01), "channel length"=[], "group index"=0, "group refnums"=[], "file name"="", "segment index"=0} ("append info out")] -> w390
                disable-tunnel: w389 -> [w413 _]
                disable-tunnel: w388 -> [w412 _]
                disable-tunnel: w387 -> [w411 _]
                disable-tunnel: w386 -> [w410 _]
                frame condition #0 (active) {
                  n97 = case shown="False" w422 {
                    tunnel: [FALSE TRUE] -> w433
                    tunnel: [w443 w503] -> w432
                    tunnel: [w441 w508] -> w427
                    tunnel: w431 -> [w471 _]
                    tunnel: w421 -> [w456 w503]
                    tunnel: [w476 w506] -> w430
                    tunnel: [w444 w507] -> w424
                    tunnel: w429 -> [w477 _]
                    tunnel: w428 -> [w473 _]
                    tunnel: w426 -> [w470 w507]
                    tunnel: [w442 w504] -> w425
                    tunnel: w420 -> [_ w501]
                    tunnel: [w457 w502] -> w423
                    tunnel: w419 -> [w464 _]
                    tunnel: w418 -> [w454 w499]
                    tunnel: [w458 _] -> w417
                    tunnel: w416 -> [w457 w502]
                    tunnel: [w454 w497] -> w415
                    tunnel: [w440 w496] -> w414
                    tunnel: w413 -> [w439 w496]
                    tunnel: w412 -> [w453 _]
                    tunnel: w411 -> [w438 _]
                    tunnel: w410 -> [w434 _]
                    frame False {
                      # "Multi file?"
                      # "New file?"
                      # "False: normal case"
                      # "serial #"
                      n98 = Unbundle By Name(w454) -> ("multi_file"=w446:bool, "new file options"=w460:T5, "new_file"=w459:bool)
                      n99 = Unbundle By Name(w454) -> ("file params"=w463:T3, "column headings"=w462:enum32{"one per segment", "once", "none"}, "origin time"=w455:timestamp)
                      n100 = case "Start a new file?" shown="True" w446 {
                        tunnel: [FALSE ("start new file?") w495] -> w472
                        tunnel: w457 -> [_ w494]
                        tunnel: w471 -> [_ w493]
                        tunnel: w460 -> [_ w492]
                        tunnel: w459 -> [_ w491]
                        frame False {
                        }
                        frame True {
                          n101 = call <vilib>:"ex_CheckMultifileTermCond.vi"("file size (bytes)"=w493, "new_file_now"=w491, "termination conditions"=w492, "Signals"=w494) -> ("start new file?"=w495:bool)  [unwired: 7 out]
                        }
                      }
                      n102 = Increment(x=w477) -> (x+1=w478:i32)
                      n103 = local read "1st"() -> (w445:bool)
                      n104 = Select(t=w478, s=w472, f=w477) -> (s? t:f=w475:i32)
                      n105 = To Long Integer(number=w475) -> (32bit integer=w476:i32)
                      n106 = Or(x=w445, y=w472) -> (x .or. y?=w447:bool)
                      n107 = Equal?(x=w462, y=enum16{"one per segment", "once", "none"}."one per segment") -> (x = y?=w466:bool)
                      n108 = case shown="True" w472 {
                        tunnel: w476 -> [_ w489]
                        tunnel: [w479 w488] -> w448
                        tunnel: w473 -> [w479 _]
                        tunnel: w470 -> [_ w487]
                        tunnel: w454 -> [_ w484]
                        frame False {
                          # "No new file - use old file name"
                        }
                        frame True {
                          # "new multi file name required"
                          n109 = Unbundle By Name(w484) -> ("serno_digits"=w483:i32, "fixed_width"=w482:bool, "new_file_mode"=w481:u16, "time_format_string"=w480:string)
                          n110 = Select(t=w483, s=w482, f=0) -> (s? t:f=w485:i32)
                          n111 = call <vilib>:"ex_BuildFilepath.vi"("serial digits"=w485, "serial num"=w489, "time format string"=w480, "naming mode"=w481, "name base"=w487) -> ("built name"=w488:path)  [unwired: 1 in, 5 out]
                        }
                      }
                      n112 = Unbundle By Name(w463) -> ("Flags"=w468:T4)
                      n113 = Bundle By Name(cluster=w468, "col headings always?"=w466) -> (w469:T4)
                      n114 = Unbundle By Name(w454) -> ("File refnum"=w458:refnum<file>, "overwrite_mode_multi"=w451:T6, "overwrite_mode"=w450:T1, "File Dialog"=w461:bool, "Description Out"=w436:string, "Comment Out"=w435:string, "Simulate Non-First Call"=w437:bool)
                      n115 = Bundle By Name(cluster=w463, "origin time"=w455, "Flags"=w469, "Flags.x_columns"=w453) -> (w452:T3)
                      n116 = Or(x=w445, y=w464) -> (x .or. y?=w465:bool)
                      n117 = And(x=w461, y=w465) -> (x .and. y?=w449:bool)
                      n118 = call <vilib>:"ex_WriteDataTDMS.vi"("file path"=w448, "first call"=w445, "Lock file"=w434, "Signals"=w457, "overwrite_mode_multi"=w451, "overwrite_mode"=w450, "error in (no error)"=w456, "file dialog?"=w449, "Description"=w436, "multi_file"=w446, "Comment"=w435, "new file?"=w447, "Simulate Non-First Call"=w437, "file params"=w452, "append info in"=w439, "DAQmx Task"=w438) -> ("operator cancelled?"=w442:bool, "file path out"=w444:path, "bytes written"=w441:i32, "append info out"=w440:T13, "error out"=w443:errorcluster)  [unwired: 7 in]
                    }
                    frame True {
                      w504 = FALSE  # operator cancelled?
                      w508 = 0  # mark after write (bytes)
                      w506 = 0  # 1st Serial #
                      # "True: First enabled call"
                      n119 = for {
                        tunnel: w501 -> [w510] mode=indexing
                        tunnel: [w509] -> w500 mode=indexing
                        n120 = Unbundle By Name(w510) -> ("Start Timestamp"=w509:timestamp)
                      }
                      n121 = Array Max & Min(array=w500) -> (min value=w498:timestamp)  [unwired: 3 out]
                      n122 = Bundle By Name(cluster=w499, "origin time"=w498) -> (w497:T11)
                    }
                  }
                }
                frame condition #1 {
                  n123 = Unbundle By Name(w518) -> ("File refnum"=w517:refnum<file>)
                }
              }
            }
          }
          n124 = case shown="True" w96 {
            tunnel: [FALSE ("Ask each iteration") "Ask each iteration"] -> w95
            frame False {
              # "Otherwise, after ex_subFileWriter.vi is invoked for the first time, set \"1st\" to false."
            }
            frame True {
              # "If \"Ask user to choose file\" is checked and \"Ask each iteration\" is selected by user, then each invocation of ex_subFileWrite.vi is treated as the first time's invocation."
            }
          }
          n125 = case shown="True" w95 {
            tunnel: w94 -> [w134 _]
            tunnel: [w134 FALSE ("operator cancelled?")] -> w93
            frame False {
            }
            frame True {
            }
          }
        }
        n126 = local write "File refnum"(w86) -> ()
        n127 = local write "1st"(w78) -> ()
        "previous path" <- w80
      }
    }
  }
  "error out" <- w30
  "File Path out" <- w29
  n128 = Not A Number/Path/Refnum?(number/path/refnum=w29) -> (NaN/Path/Refnum?=w42:bool)
  n129 = Not(x=w42) -> (.not. x?=w41:bool)
  n130 = And(x=w41, y="Enable") -> (x .and. y?=→"Saving Data":bool)
